vi "Check Status.vi"(8 "error in (no error)":errorcluster, 11 "Level Meter in":refnum<class "Level Meter.lvclass">) -> (0 "error out":errorcluster, 1 "Status":string, 2 "On?":bool, 3 "Level Meter out":refnum<class "Level Meter.lvclass">)   [LabVIEW 2009, in "Level Meter.lvclass"]
uses:
  Level Meter.lvclass
  Cryogen Levels.ctl
  Level Meter.lvclass/Level Meter.ctl
panel:
  out "cryolevels":T1 min=-1.0 max=100.0 scale=0.0..100.0
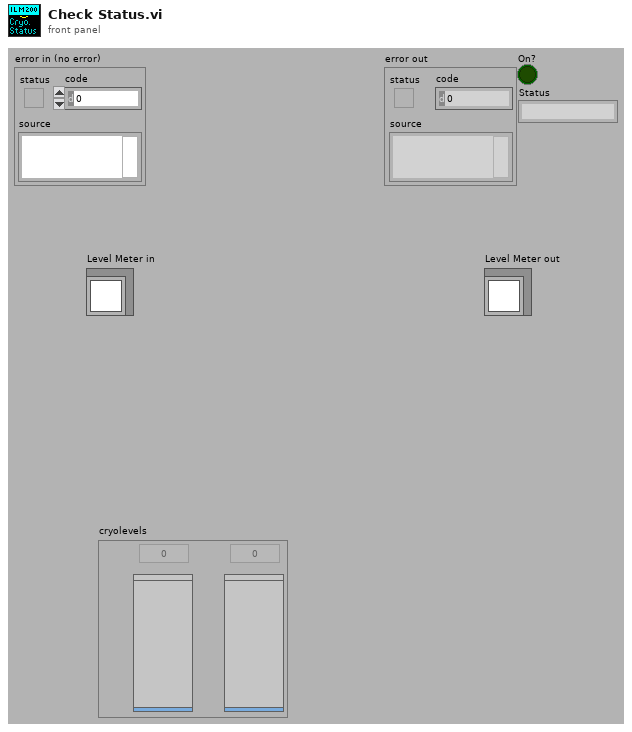
[diagram p1: front panel]
types:
  T1 = typedef "Level Meter.lvclass/Cryogen Levels.ctl" = dbl[]
  T2 = typedef "OxfordAddress.ctl" = cluster{"Com Port":i32, "ISOBUS Address":i32, "GPIB Address":i16, "Communication":enum16{"RS232", "ISOBUS", "GPIB", "Gateway"}}
  T3 = typedef "Readable.lvclass/X array.ctl" = T4[]
  T4 = typedef "Readable.lvclass/X.ctl" = dbl
  T5 = typedef "ILMRelayStatus.ctl" = cluster{"Shut down":bool, "Alarm sound":bool, "Alarm state":bool, "Silence prohib":bool, "Relay1 active":bool, "Relay 2 active":bool, "Relay 3 active":bool, "Relay 4 active":bool}
  T6 = typedef "ILMChannelStatus.ctl" = cluster{"Probe current":bool, "Probe fast":bool, "Probe slow":bool, "Auto-fill":enum16{"End fill", "Not filling", "Filling", "Start filling"}, "Fill":bool, "Low level":bool, "Alm requested":bool, "Pre-pulse I":bool}
  T7 = cluster{bool, bool, "Fill":bool, "Low level":bool}
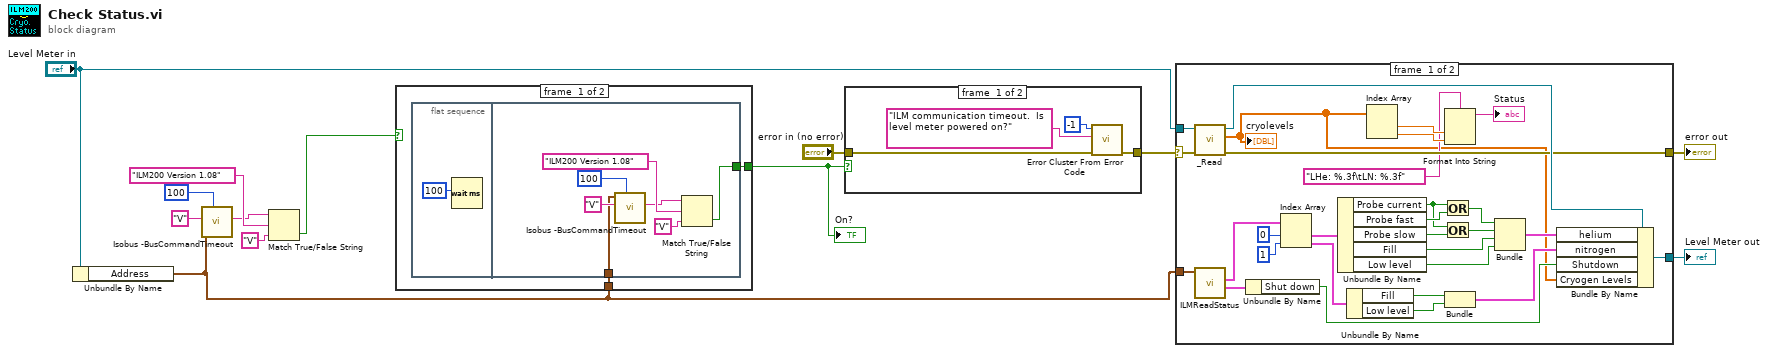
[diagram p0: block diagram]
diagram:
  n1 = Unbundle By Name("Level Meter in") -> ("Address"=w3:T2)
  n2 = call "Isobus -BusCommandTimeout.vi"("Timeout (ms)"=100, "Command"="V", "Address"=w3) -> ("Reply"=w7:string)  [unwired: 5 out]
  n3 = Match True/False String(2:"V", 3:"ILM200 Version 1.08", 4:w7) -> (0:w1:bool)  [unwired: 1 out]
  n4 = case shown="False" w1 {
    selector: w1 -> [_ w24]
    tunnel: w3 -> [w15 _]
    tunnel: [w14 w24] -> w2
    frame #0 {
      n5 = flat-sequence {
        tunnel: w15 -> [w18]
        tunnel: [w17] -> w14
        frame #0 {
          n6 = Wait (ms)(milliseconds to wait=u32 100) -> ()  [unwired: 1 out]
        }
        frame #1 {
          n7 = call "Isobus -BusCommandTimeout.vi"("Timeout (ms)"=100, "Command"="V", "Address"=w18) -> ("Reply"=w19:string)  [unwired: 5 out]
          n8 = Match True/False String(2:"V", 3:"ILM200 Version 1.08", 4:w19) -> (0:w17:bool)  [unwired: 1 out]
        }
      }
    }
    frame #1 {
    }
  }
  "On?" <- w2
  n9 = case shown="False" w2 {
    tunnel: "error in (no error)" -> [w27 w29]
    tunnel: [w26 w29] -> w4
    frame #0 {
      n10 = call <vilib>:"Error Cluster From Error Code.vi"("error in (no error)"=w27, "error message (\"\")"="ILM communication timeout.  Is level meter powered on?" ("error message (\"\")"), "error code (0)"=-1) -> ("error out"=w26:errorcluster)  [unwired: 6 in]
    }
    frame #1 {
    }
  }
  n11 = case shown="No Error" w4 {
    selector: w4 -> [w30 w59]
    tunnel: [w43 w60] -> w13
    tunnel: [w38 w59] -> w12
    tunnel: "Level Meter in" -> [w32 w60]
    tunnel: w3 -> [w31 _]
    frame #0 {
      n12 = call-dynamic "_Read.vi"("error in (no error)"=w30, "Level Meter in"=w32) -> ("error out"=w38:errorcluster, "X array"=w33:T3, "Level Meter out"=w39:refnum<class "Level Meter.lvclass">)  [unwired: 7 in]
      "cryolevels" <- w33
      n13 = call "ILMReadStatus.vi"("Instrument address"=w31) -> ("Relay"=w44:T5, "Channel"=w58:T6[])  [unwired: 5 out]
      n14 = Unbundle By Name(w44) -> ("Shut down"=w40:bool)
      n15 = Index Array(array=w58, index #1=0, index #2=1) -> (element #1=w55:T6, element #2=w54:T6)
      n16 = Unbundle By Name(w55) -> ("Probe current"=w51:bool, "Probe fast"=w52:bool, "Probe slow"=w53:bool, "Fill"=w47:bool, "Low level"=w49:bool)
      n17 = Unbundle By Name(w54) -> ("Fill"=w46:bool, "Low level"=w45:bool)
      n18 = Index Array(array=w33) -> (element #1=w37:T4, element #2=w36:T4)  [unwired: 2 in]
      n19 = Or(x=w51, y=w52) -> (x .or. y?=w50:bool)
      n20 = Or(x=w51, y=w53) -> (x .or. y?=w48:bool)
      n21 = Format Into String(format string="LHe: %.3f\tLN: %.3f", w37, w36) -> (resulting string=→"Status":string)  [unwired: 2 in, 1 out]
      n22 = Bundle("Fill"=w46, "Low level"=w45) -> (w41:cluster{"Fill":bool, "Low level":bool})  [unwired: 1 out]
      n23 = Bundle(w50, w48, "Fill"=w47, "Low level"=w49) -> (w42:T7)  [unwired: 1 out]
      n24 = Bundle By Name(cluster=w39, "helium"=w42, "nitrogen"=w41, "Shutdown"=w40, "Cryogen Levels"=w33) -> (w43:refnum<class "Level Meter.lvclass">)
    }
    frame #1 {
    }
  }
  "Level Meter out" <- w13
  "error out" <- w12
